vi "Jrk-G2_setTarget_Demo.vi"(2 "TargetValue":u16(slide)=117 scale=1448.0..2648.0, 3 "VISA Resource Name Out":refnum<visa-resource-name>="COM5") -> (0 "error out":errorcluster, 1 "Sent String":string="À@")   [LabVIEW 2020]
uses:
  Program Files (x86)/National Instruments/LabVIEW 2020/examples/Instrument IO/Serial/support/Serial - Settings.ctl
  <vilib>/Instr/_visa.llb/VISA Configure Serial Port (Instr).vi
panel:
  out "Error":bool
  out "Running":bool
  in  "Stop Motor":bool
  in  "JrkG2 Serial Settings":T1={"baud rate"=9600, "data bits"=8, "parity"=enum."None", "stop bits"=10, "flow control"=0} {"flow control" items=["None"=0, "XON/XOFF"=1, "RTS/CTS"=2, "DTR/DSR"=4]; "stop bits" items=["1.0"=10, "1.5"=15, "2.0"=20]; "data bits" min=5 max=8 step=1; "baud rate" items=["75"=75, "110"=110, "134"=134, "150"=150, "300"=300, "600"=600, "1200"=1200, "1800"=1800, "2400"=2400, "4800"=4800, "7200"=7200, "9600"=9600, "14400"=14400, "19200"=19200, "28800"=28800, "38400"=38400, "56000"=56000, "57600"=57600, "115200"=115200, "128000"=128000, "230400"=230400]}
  in  "JrkG2 VISA Port":refnum<visa-resource-name>="COM5"
  out "Target_Cmd":u16=192 format="%x"
  out "Target_Val":u16=64 format="%x"
  # "Input:\nSerial Port JrkG2 is connected to.\n(Disabled in Standalone Mode)"
  # "Serial Port Setup\n(For use in Standalone Mode)"
  # "Moving the Motor connected to the Jrk G2. \n(Controls speed in a direction)"
  # "Output for Serial Commands:"
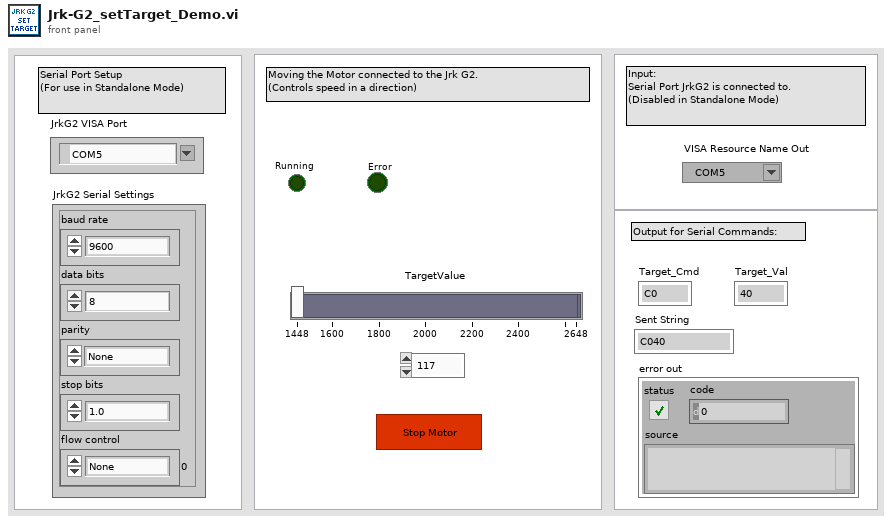
[diagram p1: front panel]
types:
  T1 = typedef "Serial - Settings.ctl" = cluster{"baud rate":u32, "data bits":u16, "parity":enum16{"None", "Odd", "Even", "Mark", "Space"}, "stop bits":u16, "flow control":u16}
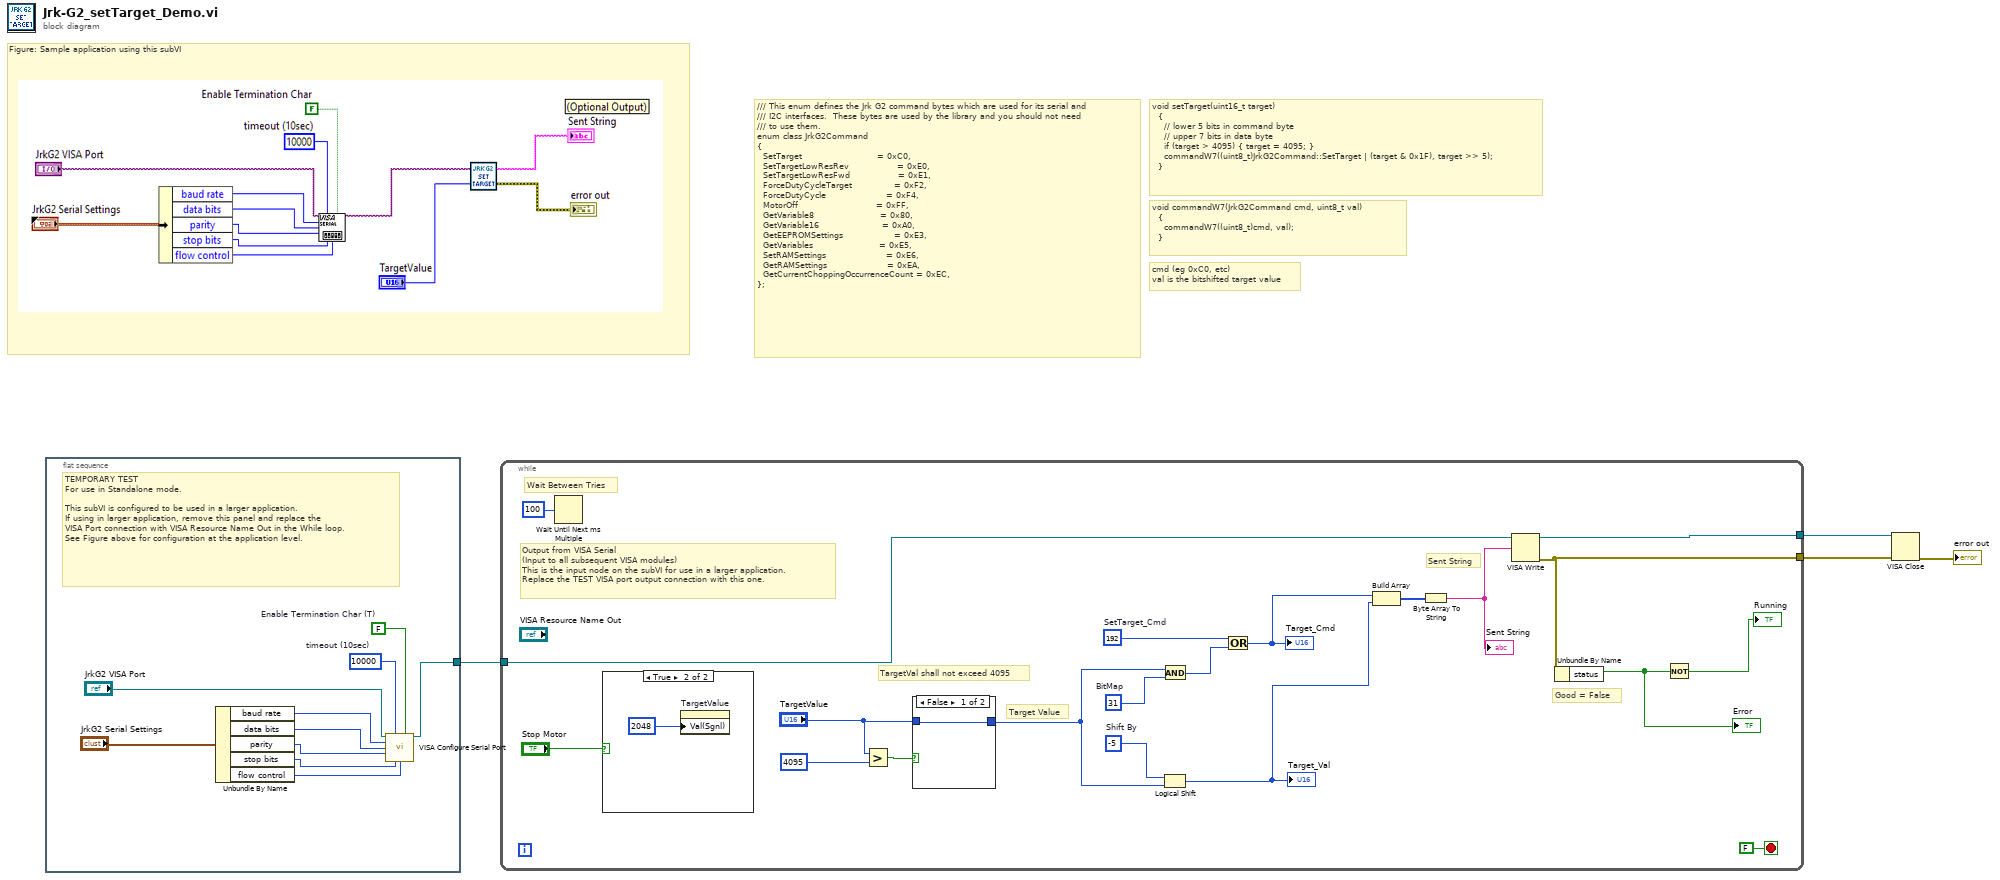
[diagram p0: block diagram]
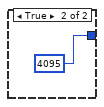
[diagram p3: hidden frame]
diagram:
  # "void commandW7(JrkG2Command cmd, uint8_t val)\n  {\n    commandW7((uint8_t)cmd, val);\n  }"
  # "cmd (eg 0xC0, etc)\nval is the bitshifted target value"
  # "void setTarget(uint16_t target)\n  {\n    // lower 5 bits in command byte\n    // upper 7 bits in data byte\n    if (target > 4095) { target = 4095; }\n    commandW7((uint8_t)JrkG2Command::SetTarget | (target & 0x1F), target >> 5);\n  }"
  # "/// This enum defines the Jrk G2 command bytes which are used for its serial and\n/// I2C interfaces.  These bytes are used by the library and you should not need\n/// to use them.\nenum class JrkG2Command\n{\n  SetTarget                         = 0xC0,\n  SetTargetLowResRev                = 0xE0,\n  SetTargetLowResFwd                = 0xE1,\n  ForceDutyCycleTarget              = 0xF2,\n  ForceDutyCycle                    = 0xF4,\n  MotorOff                          = 0xFF,\n  GetVariable8                      = 0x80,\n  GetVariable16                     = 0xA0,\n  GetEEPROMSettings                 = 0xE3,\n  GetVariables                      = 0xE5,\n  SetRAMSettings                    = 0xE6,\n  GetRAMSettings                    = 0xEA,\n  GetCurrentChoppingOccurrenceCount = 0xEC,\n};"
  # "Figure: Sample application using this subVI"
  n1 = flat-sequence {
    tunnel: [w5] -> w1
    frame #0 {
      w6 = u32 10000  # timeout (10sec)
      w7 = FALSE  # Enable Termination Char (T)
      # "TEMPORARY TEST \nFor use in Standalone mode.\n\nThis subVI is configured to be used in a larger application.\nIf using in larger application, remove this panel and replace the \nVISA Port connection with VISA Resource Name Out in the While loop.\nSee Figure above for configuration at the application level."
      n2 = Unbundle By Name("JrkG2 Serial Settings") -> ("baud rate"=w13:u32, "data bits"=w12:u16, "parity"=w11:enum16{"None", "Odd", "Even", "Mark", "Space"}, "stop bits"=w10:u16, "flow control"=w9:u16)
      n3 = call-poly "VISA Configure Serial Port"("VISA resource name"="JrkG2 VISA Port", "timeout (10sec)"=w6, "Enable Termination\nChar (T)"=w7, "baud rate (9600)"=w13, "data bits (8)"=w12, "parity (0:none)"=w11, "stop bits (10: 1 bit)"=w10, "flow control (0:none)"=w9) -> ("VISA resource name out"=w5:refnum<visa-resource-name>)  [unwired: 1 in, 6 out]
    }
  }
  n4 = while {
    tunnel: [w26] -> w4
    tunnel: [w25] -> w3
    tunnel: w1 -> [w20]
    stop <- FALSE stop-if-true
    w29 = -5  # Shift By
    w32 = u16 31  # BitMap
    w30 = u16 192  # SetTarget_Cmd
    # "Good = False"
    # "Wait Between Tries"
    # "Sent String"
    # "Output from VISA Serial\n(Input to all subsequent VISA modules)\nThis is the input node on the subVI for use in a larger application.  \nReplace the TEST VISA port output connection with this one."
    # "Target Value"
    # "TargetVal shall not exceed 4095"
    n5 = Wait Until Next ms Multiple(millisecond multiple=100) -> ()  [unwired: 1 out]
    n6 = case shown="True" "Stop Motor" {
      frame False {
      }
      frame True {
        n7 = property on="TargetValue" class="Slide (strict)"("Val(Sgnl)"=u16 2048 ("Value (Signaling)")) -> ()  [unwired: 2 in, 2 out]
      }
    }
    n8 = Greater?(x="TargetValue", y=u16 4095) -> (0:w34:bool)
    n9 = case shown="False" w34 {
      tunnel: "TargetValue" -> [w36 _]
      tunnel: [w36 u16 4095 ("y")] -> w28
      frame False {
      }
      frame True {
      }
    }
    n10 = Logical Shift(y=w29, x=w28) -> (x << y=w21:u16)
    "Target_Val" <- w21
    n11 = And(x=w28, y=w32) -> (x .and. y?=w31:u16)
    n12 = Or(x=w30, y=w31) -> (x .or. y?=w22:u16)
    "Target_Cmd" <- w22
    n13 = Build Array(w22, w21) -> (w23:u16[])
    n14 = Byte Array To String(unsigned byte array=w23) -> (string=w27:string)
    "Sent String" <- w27
    n15 = VISA Write(VISA resource name=w20, write buffer=w27) -> (VISA resource name out=w26:refnum<visa-resource-name>, error out=w25:errorcluster)  [unwired: 1 in, 1 out]
    n16 = Unbundle By Name(w25) -> ("status"=w16:bool)
    "Error" <- w16
    n17 = Not(x=w16) -> (.not. x?=→"Running":bool)
  }
  n18 = VISA Close(VISA resource name=w4, error in (no error)=w3) -> (error out=→"error out":errorcluster)
